vi "Channels.vi"   [LabVIEW 2018, in "OXYGEN.lvlib"]
uses:
  OXYGEN.lvlib
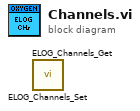
[diagram p0: block diagram]
diagram:
  n1 = call "ELOG_Channels_Set.vi"() -> ()  [unwired: 9 in, 3 out]
  n2 = call "ELOG_Channels_Get.vi"() -> ()  [unwired: 8 in, 4 out]
